vi "ShiftReg Test 1.vi"() -> ()   [LabVIEW 2014]
panel:
  out "Array 3":i32[](array[numeric])
  out "Array 2":i32[](array[numeric])
  out "Array":i32[](array[numeric])
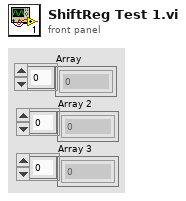
[diagram p1: front panel]
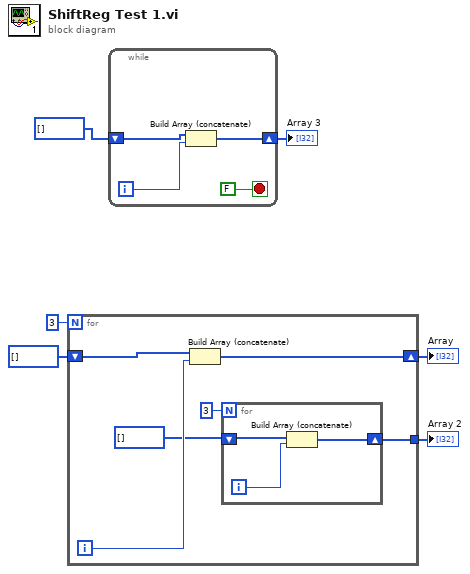
[diagram p0: block diagram]
diagram:
  n1 = for {
    N: 3 -> [_]
    shift-right: [w10] -> w5
    shift-left: i32[] [] -> [w11]
    tunnel: [w8] -> w4
    i -> [w12]
    n2 = Build Array (concatenate)(w11, w12) -> (w10:i32[])
    n3 = for {
      N: 3 -> [_]
      shift-right: [w14] -> w8
      shift-left: i32[] [] -> [w15]
      i -> [w13]
      n4 = Build Array (concatenate)(w15, w13) -> (w14:i32[])
    }
  }
  "Array" <- w5
  "Array 2" <- w4
  n5 = while {
    shift-right: [w17] -> w1
    shift-left: i32[] [] -> [w18]
    i -> [w16]
    stop <- FALSE stop-if-true
    n6 = Build Array (concatenate)(w18, w16) -> (w17:i32[])
  }
  "Array 3" <- w1
